vi "AO AE.vi"(8 "Mirror Modes In":T1, 9 "DM Value Input":dbl[][](array[numeric]), 10 "Z Comp. Input":T2, 11 "Action":enum16{"READ", "WRITE"}(ring)) -> (0 "Mirror Modes Out":T1, 1 "DM Value Output":dbl[][](array[numeric]), 2 "Z Comp. Output":T2)   [LabVIEW 2014]
uses:
  Type Defs/Z comp.ctl
  DM_Dual_V2/Controls/MirrorModes_DUAL.ctl
panel:
  # "Piston"
  # "Defocus"
  # "Spherical"
  # "Piston"
  # "Defocus"
  # "Spherical"
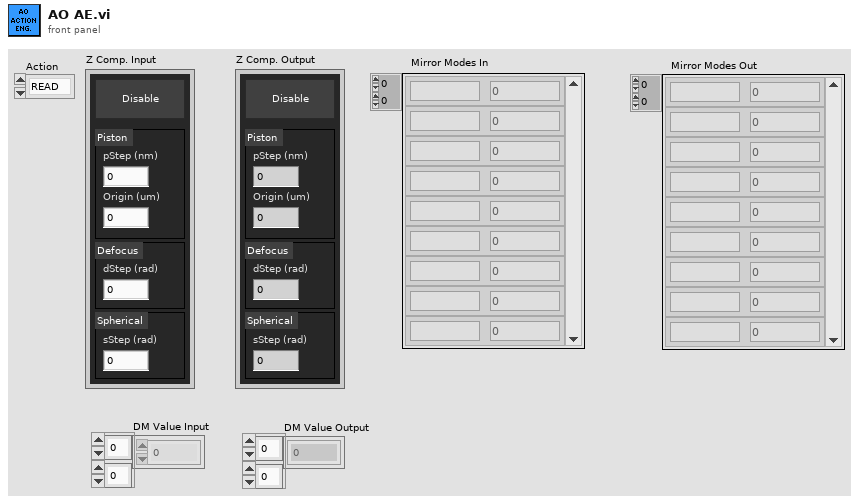
[diagram p1: front panel]
types:
  T1 = typedef "MirrorModes_DUAL.ctl" = cluster{"Mode":string, "Amplitude":dbl}[][]
  T2 = typedef "Z comp.ctl" = cluster{"Enable":bool, "pStep (nm)":dbl, "Origin (um)":dbl, "dStep (rad)":dbl, "sStep (rad)":dbl}
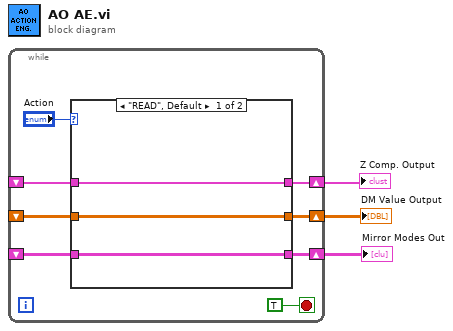
[diagram p0: block diagram]
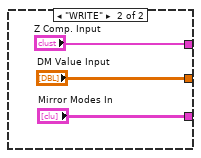
[diagram p2: hidden frame]
diagram:
  n1 = while {
    shift-right: [w9] -> w3
    shift-left: _ -> [w8]
    shift-right: [w7] -> w2
    shift-left: _ -> [w6]
    shift-right: [w5] -> w1
    shift-left: _ -> [w4]
    stop <- TRUE stop-if-true
    n2 = case shown="\"READ\", Default" "Action" {
      tunnel: [w14 "Z Comp. Input"] -> w9
      tunnel: w8 -> [w14 _]
      tunnel: [w13 "DM Value Input"] -> w7
      tunnel: w6 -> [w13 _]
      tunnel: [w12 "Mirror Modes In"] -> w5
      tunnel: w4 -> [w12 _]
      frame "READ", Default {
      }
      frame "WRITE" {
      }
    }
  }
  "Z Comp. Output" <- w3
  "DM Value Output" <- w2
  "Mirror Modes Out" <- w1
